vi "VG_VCellMin70_P.vi"() -> ()   [LabVIEW 2020]
panel:
  out "VCellMin70":dbl
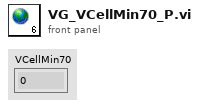
[diagram p1: front panel]
diagram:
